vi "FeedbackDecode_DEKAHandCtrl.vi"(1 "RunMode":enum16{"Manual", "Decode"}(ring)) -> ()   [LabVIEW 2020]
uses:
  FeedbackDecode_Globals.vi
  FeedbackDecode_DecodeClust.ctl
  FeedbackDecode_VariablesToString_MDArray.vi
  <vilib>/nican/nican.llb/ncNetAttr.ctl
  <vilib>/nican/nican.llb/CanFrameTimed.ctl
panel:
  in  "DEKAMode":enum16{"Velocity", "Position"}(ring)=enum."Position"
  in  "CtrlMode":T1(array[ring])=[enum."Position", enum."Position", enum."Position", enum."Position", enum."Position", enum."Position", enum."Position", enum."Position", enum."Position", enum."Position", enum."Position", enum."Position"]
  out "MinMax":dbl[][](array[numeric])=[[nan, nan, nan, nan, nan, nan, nan, nan, nan, nan, nan, nan, nan], [nan, nan, nan, nan, nan, nan, nan, nan, nan, nan, nan, nan, nan]]
  in  "Calibrate":bool
  out "LoopCnt":i32
  out "CtrlLoop":dbl(graph)
  in  "ConnDEKA":bool
  in  "MSMSMvnt":dbl[](array[numeric])=[0.0, 0.0, 0.0, 0.0, 0.0, 0.0, 0.0, 0.0, 0.0, 0.0, 0.0, 0.0] min=-1.0 max=1.0
  in  "SensorsRaw":T2={"x241"=[0, 0, 0, 0, 0, 0, 0, 0], "x341"=[0, 0, 0, 0, 0, 0, 0, 0], "x4C2"=[0, 0, 0, 0, 0, 0, 0, 0], "x4AA"=[0, 0, 0, 0, 0, 0, 0, 0], "x4BF"=[0, 0, 0, 0, 0, 0, 0, 0]}
  out "ACITime":dbl(graph)
  out "ACIs":T3[](array[typedef])=[{"Timestamp"=0.0, "ArbitrationId"=528, "IsRemote"=0, "DataLength"=8, "Data"=[0, 0, 0, 0, 0, 0, 0, 0]}, {"Timestamp"=0.0, "ArbitrationId"=529, "IsRemote"=0, "DataLength"=8, "Data"=[0, 0, 0, 0, 0, 0, 0, 0]}, {"Timestamp"=0.0, "ArbitrationId"=530, "IsRemote"=0, "DataLength"=8, "Data"=[0, 0, 0, 0, 0, 0, 0, 0]}, {"Timestamp"=0.0, "ArbitrationId"=531, "IsRemote"=0, "DataLength"=8, "Data"=[0, 0, 0, 0, 0, 0, 0, 0]}] {"Data" format="%.0x"; "ArbitrationId" format="%.0x"; "Timestamp" format="%<%I:%M:%S%3u %p\n%m/%d/%Y>T"}
  out "Sensors":T4
  in  "index":i32
  out "SensorChart":dbl(graph)=12.0
  out "LoopTime":dbl(graph)
  in  "CANConfig":T5={"Start On Open"=enum."TRUE", "Baud Rate"=1000000, "Read Queue Length"=100, "Write Queue Length"=12, "Standard Comparator"=0, "Standard Mask"=0, "Extended Comparator"=0, "Extended Mask"=0} {"Baud Rate" min=5000 max=1333333 step=1; "Extended Mask" format="%.0x"; "Extended Comparator" format="%.0x"; "Standard Mask" format="%.0x"; "Standard Comparator" format="%.0x"; "Write Queue Length" max=1000; "Read Queue Length" max=1000}
  out "Error out":errorcluster {"code" format="%.0x"}
  in  "stop":bool
  in  "CANport":string="CAN0"
  # "ThuPitchUp"
  # "ThuPitchDown"
  # "ThuYawRight"
  # "ThuYawLeft"
  # "IndFlex"
  # "IndExt"
  # "MRPFlex"
  # "MRPExt"
  # "WriPronate"
  # "WriSupinate"
  # "WriExt"
  # "WriFlex"
  # "ModeSelect"
  # "N/A"
  # "N/A"
  # "N/A"
  # "Thumb"
  # "Index"
  # "Middle"
  # "Ring"
  # "Little"
  # "ThumbInt"
  # "IndexInt"
  # "Ring Int"
  # "Little Int"
  # "WristPitch"
  # "WristYaw"
  # "WristRoll"
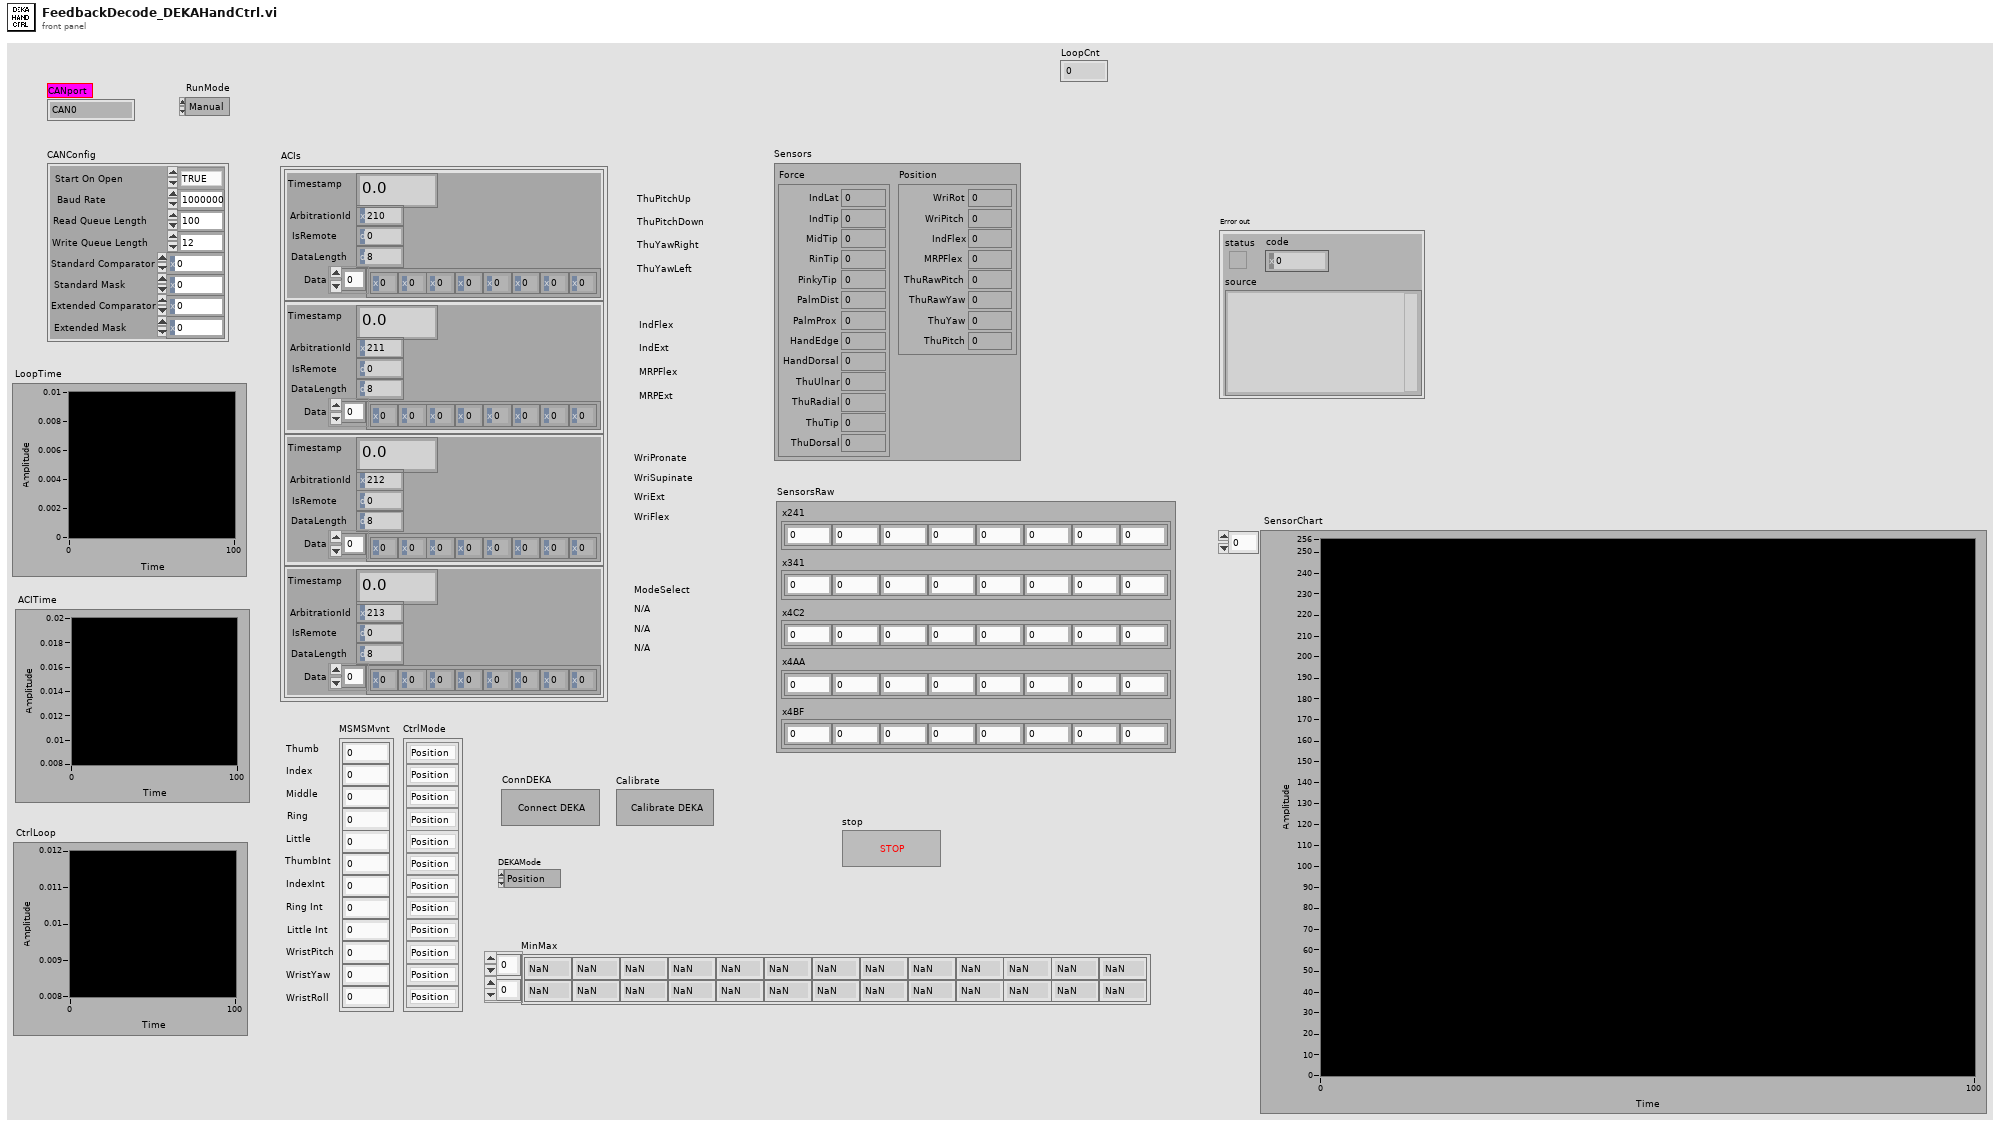
[diagram p1: front panel]
types:
  T1 = enum16{"Position", "Latching", "Leaky", "Velocity"}[]
  T2 = cluster{"x241":u8[], "x341":u8[], "x4C2":u8[], "x4AA":u8[], "x4BF":u8[]}
  T3 = typedef "CanFrameTimed.ctl" = cluster{"Timestamp":dbl, "ArbitrationId":u32, "IsRemote":u8, "DataLength":u8, "Data":u8[]}
  T4 = cluster{"Position":cluster{"WriRot":dbl, "WriPitch":dbl, "IndFlex":dbl, "MRPFlex":dbl, "ThuRawPitch":dbl, "ThuRawYaw":dbl, "ThuYaw":dbl, "ThuPitch":dbl}, "Force":cluster{"IndLat":dbl, "IndTip":dbl, "MidTip":dbl, "RinTip":dbl, "PinkyTip":dbl, "PalmDist":dbl, "PalmProx":dbl, "HandEdge":dbl, "HandDorsal":dbl, "ThuUlnar":dbl, "ThuRadial":dbl, "ThuTip":dbl, "ThuDorsal":dbl}}
  T5 = typedef "ncNetAttr.ctl" = cluster{"Start On Open":enum32{"FALSE", "TRUE"}, "Baud Rate":u32, "Read Queue Length":u32, "Write Queue Length":u32, "Standard Comparator":u32, "Standard Mask":u32, "Extended Comparator":u32, "Extended Mask":u32}
  T6 = typedef "xobjhandle.ctl" = u32
  T7 = enum16{"Position", "Latching", "Leaky", "Velocity"}
  T8 = typedef "FeedbackDecode_DecodeClust.ctl" = cluster{"TrainParams":cluster{"Lag":dbl, "KernelWidth":dbl, "TargRad":dbl}, "Kinematics":cluster{"Thumb":dbl, "Index":dbl, "Middle":dbl, "Ring":dbl, "Little":dbl, "ThumbInt":dbl, "IndexInt":dbl, "RingInt":dbl, "LittleInt":dbl, "Wrist":dbl, "WristYaw":dbl, "WristRoll":dbl}, "CtrlButtons":cluster{"AcqTraining":bool, "ApplyBaseline":bool, "ApplyTraining":bool, "LoadTrainFile":bool, "CAR":bool, "NIPSpikes":bool, "AcqBaseline":bool, "Stop":bool, "ResetTrial":bool, "CalDEKA":bool, "HideSphrs":bool, "StartTrials":bool, "AutoPop":bool, "ResetVRE":bool, "StopVRE":bool, "AcqCAR":bool, "ConARD":bool, "DEKARestart":bool, "ConnDEKA":bool}, "CompID":cluster{"LV":cluster{"Name":string, "IP":string}, "ML":cluster{"Name":string, "IP":string}}, "KMvntClust":cluster{"KGain":sgl[][], "KMvnts":cluster{"Thumb":bool, "Index":bool, "Middle":bool, "Ring":bool, "Little":bool, "ThumbInt":bool, "IndexInt":bool, "RingInt":bool, "LittleInt":bool, "WristPitch":bool, "WristYaw":bool, "WristRoll":bool}, "KThresh":sgl[][], "CtrlMode":enum16{"Position", "Latching", "Leaky", "Velocity"}[], "CtrlSpd":sgl[]}, "ClearUEA":bool, "Targets":cluster{"Thumb":dbl, "Index":dbl, "Middle":dbl, "Ring":dbl, "Little":dbl, "ThumbInt":dbl, "IndexInt":dbl, "RingInt":dbl, "LittleInt":dbl, "Wrist":dbl, "WristYaw":dbl, "WristRoll":dbl}, "KUEAArray":cluster{"Boolean 1":bool, "Boolean 2":bool, "Boolean 3":bool, "Boolean 4":bool, "Boolean 5":bool, "Boolean 6":bool, "Boolean 7":bool, "Boolean 8":bool, "Boolean 9":bool, "Boolean 10":bool, "Boolean 11":bool, "Boolean 12":bool, "Boolean 13":bool, "Boolean 14":bool, "Boolean 15":bool, "Boolean 16":bool, "Boolean 17":bool, "Boolean 18":bool, "Boolean 19":bool, "Boolean 20":bool, "Boolean 21":bool, "Boolean 22":bool, "Boolean 23":bool, "Boolean 24":bool, "Boolean 25":bool, "Boolean 26":bool, "Boolean 27":bool, "Boolean 28":bool, "Boolean 29":bool, "Boolean 30":bool, "Boolean 31":bool, "Boolean 32":bool, "Boolean 33":bool, "Boolean 34":bool, "Boolean 35":bool, "Boolean 36":bool, "Boolean 37":bool, "Boolean 38":bool, "Boolean 39":bool, "Boolean 40":bool, "Boolean 41":bool, "Boolean 42":bool, "Boolean 43":bool, "Boolean 44":bool, "Boolean 45":bool, "Boolean 46":bool, "Boolean 47":bool, "Boolean 48":bool, "Boolean 49":bool, "Boolean 50":bool, "Boolean 51":bool, "Boolean 52":bool, "Boolean 53":bool, "Boolean 54":bool, "Boolean 55":bool, "Boolean 56":bool, "Boolean 57":bool, "Boolean 58":bool, "Boolean 59":bool, "Boolean 60":bool, "Boolean 61":bool, "Boolean 62":bool, "Boolean 63":bool, "Boolean 64":bool, "Boolean 65":bool, "Boolean 66":bool, "Boolean 67":bool, "Boolean 68":bool, "Boolean 69":bool, "Boolean 70":bool, "Boolean 71":bool, "Boolean 72":bool, "Boolean 73":bool, "Boolean 74":bool, "Boolean 75":bool, "Boolean 76":bool, "Boolean 77":bool, "Boolean 78":bool, "Boolean 79":bool, "Boolean 80":bool, "Boolean 81":bool, "Boolean 82":bool, "Boolean 83":bool, "Boolean 84":bool, "Boolean 85":bool, "Boolean 86":bool, "Boolean 87":bool, "Boolean 88":bool, "Boolean 89":bool, "Boolean 90":bool, "Boolean 91":bool, "Boolean 92":bool, "Boolean 93":bool, "Boolean 94":bool, "Boolean 95":bool, "Boolean 96":bool, "Boolean 97":bool, "Boolean 98":bool, "Boolean 99":bool, "Boolean 100":bool}[], "ReTrain":bool, "TargDist":dbl[], "State":enum16{"Initialize", "Acquire Start", "Acquire Response", "Finalize"}, "KalmanType":enum16{"Standard", "Mean", "Refit", "LinSVReg", "NonLinSVReg", "PCA", "DWPRR", "AdaptKF", "NN", "NN_python", "AdaptKF2", "KF_Short_Goal"}, "EventStr":string, "SelElect":dbl, "KinSrc":enum16{"Off", "Training", "Decode", "COB", "LEAP"}, "HoverElect":dbl, "RasterWin":dbl, "WfCnt":dbl, "ClearWfs":bool, "ApplyThresh":bool, "ThreshVal":dbl, "ThreshMode":enum16{"RMS Single", "RMS All", "RMS Auto", "Volt Single", "Volt All"}, "DataFolder":string, "ClearEMG":bool, "KEMGClust":cluster{"Boolean 92":bool, "Boolean 82":bool, "Boolean 72":bool, "Boolean 62":bool, "Boolean 52":bool, "Boolean 42":bool, "Boolean 32":bool, "Boolean 22":bool, "Boolean 12":bool, "Boolean 2":bool, "Boolean 93":bool, "Boolean 83":bool, "Boolean 73":bool, "Boolean 63":bool, "Boolean 53":bool, "Boolean 43":bool, "Boolean 33":bool, "Boolean 23":bool, "Boolean 13":bool, "Boolean 3":bool, "Boolean 94":bool, "Boolean 84":bool, "Boolean 74":bool, "Boolean 64":bool, "Boolean 54":bool, "Boolean 44":bool, "Boolean 34":bool, "Boolean 24":bool, "Boolean 14":bool, "Boolean 4":bool, "Boolean 95":bool, "Boolean 85":bool, "Boolean 75":bool, "Boolean 65":bool, "Boolean 55":bool, "Boolean 45":bool, "Boolean 35":bool, "Boolean 25":bool, "Boolean 15":bool, "Boolean 5":bool, "Boolean 96":bool, "Boolean 86":bool, "Boolean 76":bool, "Boolean 66":bool, "Boolean 56":bool, "Boolean 46":bool, "Boolean 36":bool, "Boolean 26":bool, "Boolean 16":bool, "Boolean 6":bool, "Boolean 97":bool, "Boolean 87":bool, "Boolean 77":bool, "Boolean 67":bool, "Boolean 57":bool, "Boolean 47":bool, "Boolean 37":bool, "Boolean 27":bool, "Boolean 17":bool, "Boolean 7":bool, "Boolean 98":bool, "Boolean 88":bool, "Boolean 78":bool, "Boolean 68":bool, "Boolean 58":bool, "Boolean 48":bool, "Boolean 38":bool, "Boolean 28":bool, "Boolean 18":bool, "Boolean 8":bool, "Boolean 99":bool, "Boolean 89":bool, "Boolean 79":bool, "Boolean 69":bool, "Boolean 59":bool, "Boolean 49":bool, "Boolean 39":bool, "Boolean 29":bool, "Boolean 19":bool, "Boolean 9":bool}, "EvntFlag":bool, "FillUEA":bool, "FillEMG":bool, "FillMvnts":bool, "BadUEAElects":dbl[], "KEMGExtra":dbl[], "AllPairs":bool, "AutoThresh":dbl, "BadEMGChans":dbl[], "LinkedDOF":string, "AutoPopType":enum16{"Standard", "Stepwise", "Gram"}, "CARType":enum16{"Standard", "NN"}, "*Map":enum16{"pNeural/pEMG", "pNeural/aEMG", "aNeural/pEMG", "aNeural/aEMG", "N2021/pEMG"}, "GainFill":dbl, "ThreshFill":dbl, "TestType":enum16{"MSMS", "Bakeoff11", "Bakeoff21", "Bakeoff31", "Bakeoff32", "Bakeoff32_Ball", "Bakeoff32_Checkers", "Bakeoff32_Pen", "FragileBlock"}, "Outcome":enum16{"---", "Success", "Failure"}, "TrialCnt":dbl[][], "ClearTrials":bool, "Log10":bool, "KDFFile":string, "LimitExt":bool, "*Prosthesis":enum16{"MaleRight", "MaleLeft"}, "StartML":bool, "StartMLAux":bool, "StartRec":bool, "DynaThr":bool, "ModeFill":enum16{"Position", "Latching", "Leaky", "Velocity"}, "SpdFill":dbl, "DEKAMode":enum16{"Velocity", "Position"}, "FreeParam":dbl, "GoalNoise":dbl, "Load NN":bool, "ExportTrain":bool, "NumComp":enum16{"1 Computer", "2 Computers"}, "DataDir":string, "BuildDir":string, "LatchingFilter":bool, "Trigger":bool, "StartARD":bool, "StartTaska":bool, "StartTaskaSens":bool}
  T9 = enum16{"Initialize", "Wait", "BuildInitStr", "BuildKalmanStr", "BuildStimStr", "BuildEMGStr", "GetEvent", "SendEvent", "ContIO", "LoadTrainFile", "CopyTraining", "Close"}
  T10 = cluster{"IndLat":dbl, "IndTip":dbl, "MidTip":dbl, "RinTip":dbl, "PinkyTip":dbl, "PalmDist":dbl, "PalmProx":dbl, "HandEdge":dbl, "HandDorsal":dbl, "ThuUlnar":dbl, "ThuRadial":dbl, "ThuTip":dbl, "ThuDorsal":dbl}
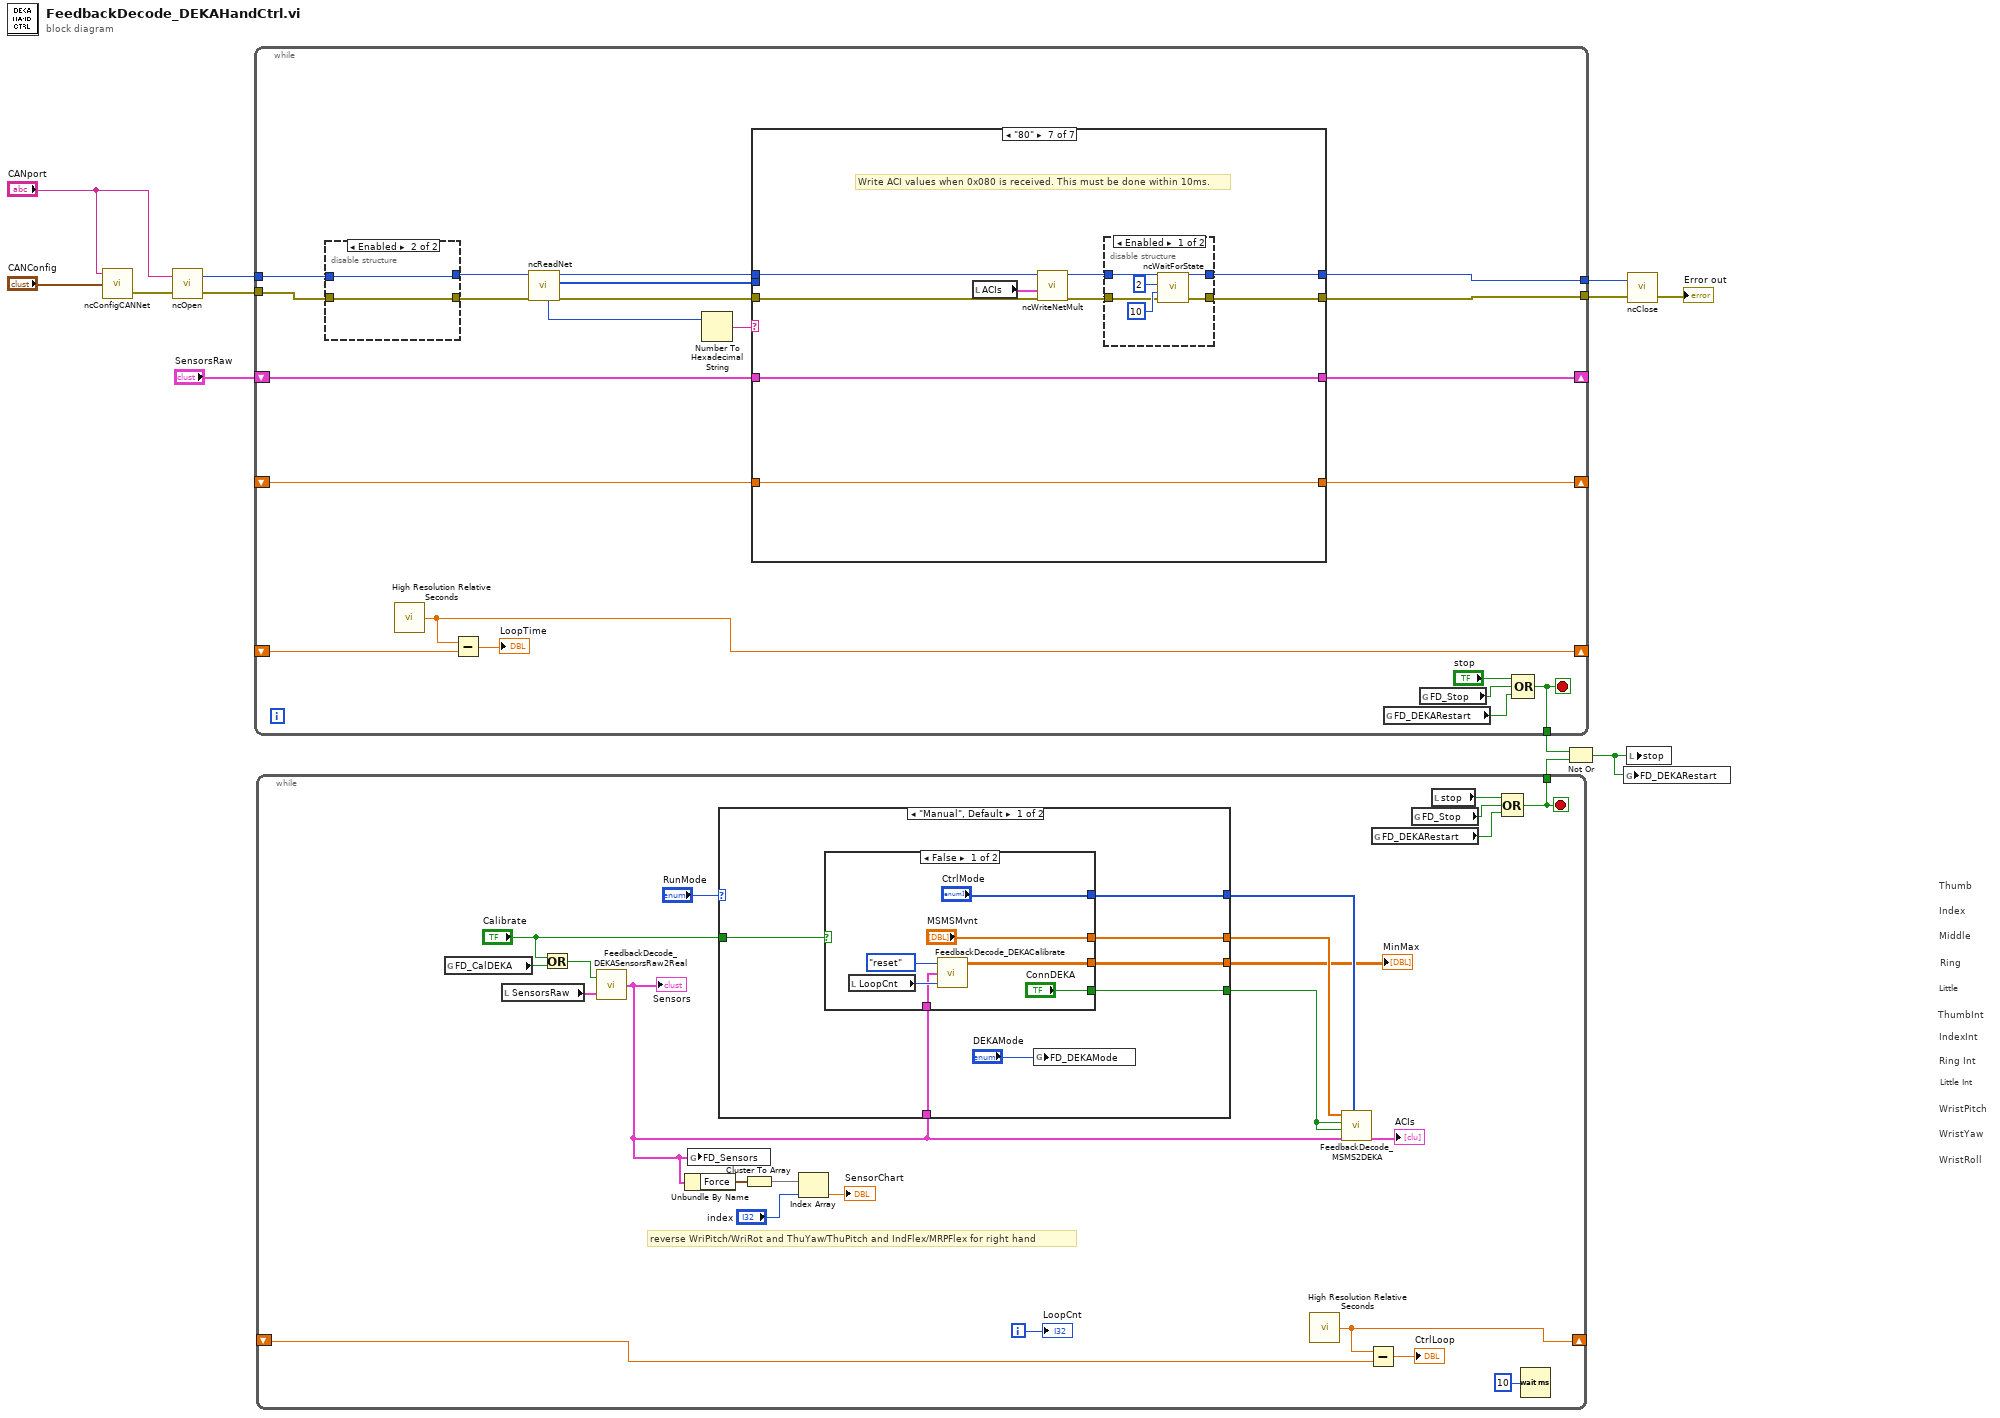
[diagram p0: block diagram]
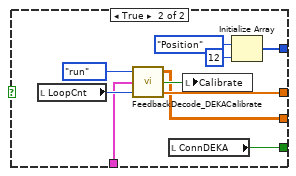
[diagram p2: hidden frame]
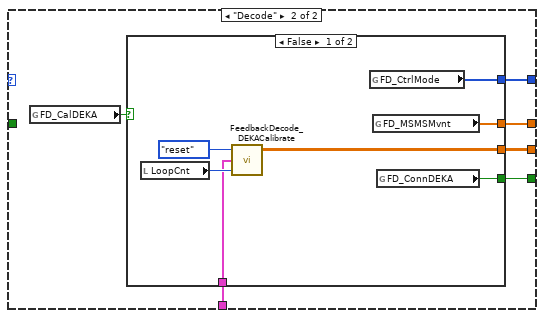
[diagram p3: hidden frame]
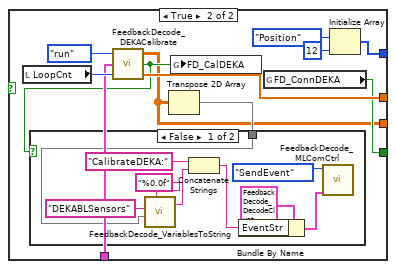
[diagram p4: hidden frame]
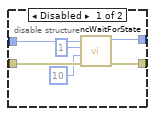
[diagram p6: hidden frame]
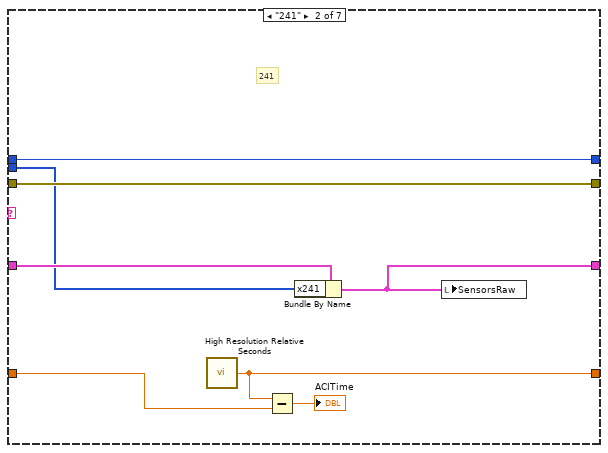
[diagram p8: hidden frame]
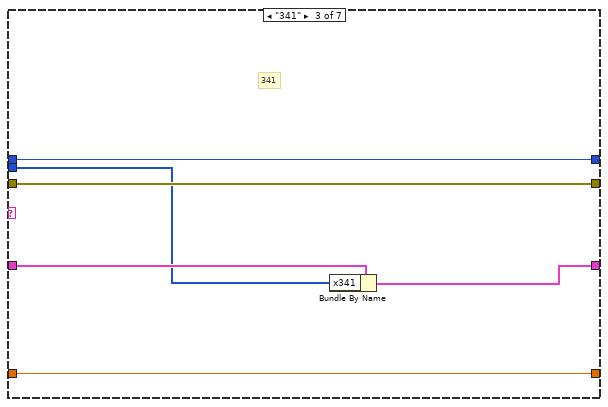
[diagram p9: hidden frame]
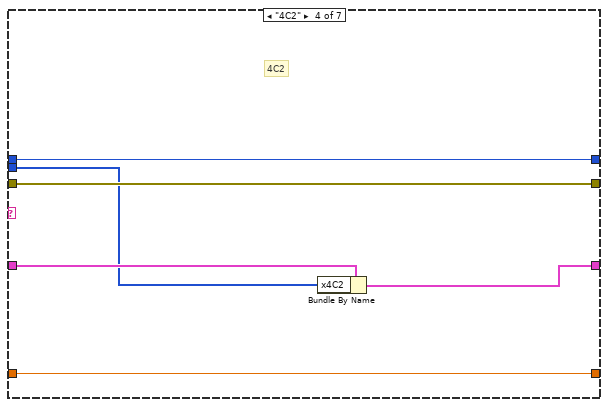
[diagram p10: hidden frame]
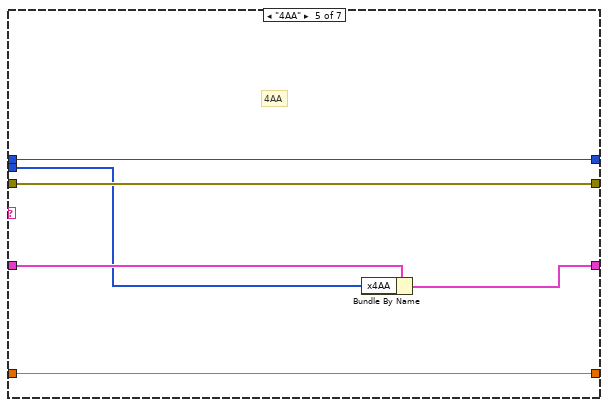
[diagram p11: hidden frame]
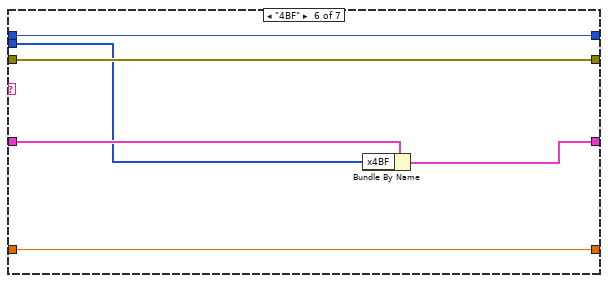
[diagram p12: hidden frame]
diagram:
  # "Little Int"
  # "WristRoll"
  # "WristYaw"
  # "WristPitch"
  # "Ring Int"
  # "IndexInt"
  # "ThumbInt"
  # "Little"
  # "Ring"
  # "Middle"
  # "Index"
  # "Thumb"
  n1 = call <vilib>:"ncConfigCANNet.vi"("CAN Network Interface Config"="CANConfig", "ObjName"="CANport") -> ("Error out"=w11:errorcluster)  [unwired: 3 in]
  n2 = call <vilib>:"ncOpen.vi"("Error in"=w11, "ObjName"="CANport") -> ("Error out"=w5:errorcluster, "ObjHandle out"=w6:T6)
  n3 = while {
    tunnel: w5 -> [w34]
    tunnel: [w25] -> w10
    tunnel: w6 -> [w32]
    tunnel: [w28] -> w8
    shift-right: [w29] -> _
    shift-left: _ -> [w30]
    shift-right: [w23] -> _
    shift-left: "SensorsRaw" -> [w24]
    shift-right: [w17] -> _
    shift-left: _ -> [w18]
    tunnel: [w14] -> w4
    stop <- w14 stop-if-true
    n4 = disable-structure shown="Enabled" {
      disable-tunnel: w34 -> [w40 w41]
      disable-tunnel: [w39 w41] -> w33
      disable-tunnel: w32 -> [w38 w42]
      disable-tunnel: [w37 w42] -> w31
      frame Disabled {
        n5 = call <vilib>:"ncWaitForState.vi"("Error in"=w40, "Timeout"=u32 10, "DesiredState"=u32 1 ("state"), "ObjHandle in"=w38) -> ("Error out"=w39:errorcluster, "ObjHandle out"=w37:T6)  [unwired: 1 out]
      }
      frame Enabled {
      }
    }
    n6 = call <vilib>:"High Resolution Relative Seconds.vi"() -> ("relative seconds"=w29:dbl)
    n7 = Subtract(x=w29, y=w30) -> (x-y=→"LoopTime":dbl)
    n8 = call <vilib>:"ncReadNet.vi"("ObjHandle in"=w31, "Error in"=w33) -> ("ArbitrationId"=w20:u32, "ObjHandle out"=w27:T6, "Data"=w19:u8[], "Error out"=w26:errorcluster)  [unwired: 2 in, 3 out]
    n9 = Number To Hexadecimal String(2:w20) -> (0:w21:string)  [unwired: 1 in]
    n10 = case shown="\"80\"" w21 {
      tunnel: [w46 w54 w60 w66 w72 w78 w82] -> w28
      tunnel: w27 -> [w46 w54 w60 w66 w72 w78 w87]
      tunnel: w19 -> [_ w51 w55 w61 w67 w73 _]
      tunnel: w26 -> [w45 w53 w59 w65 w71 w77 w86]
      tunnel: [w45 w53 w59 w65 w71 w77 w83] -> w25
      tunnel: w24 -> [w44 w52 w58 w64 w70 w76 w80]
      tunnel: [w44 w50 w57 w63 w69 w75 w80] -> w23
      tunnel: w18 -> [w43 w48 w56 w62 w68 w74 w79]
      tunnel: [w43 w47 w56 w62 w68 w74 w79] -> w17
      frame "0", Default {
      }
      frame "241" {
        # "241"
        n11 = call <vilib>:"High Resolution Relative Seconds.vi"() -> ("relative seconds"=w47:dbl)
        n12 = Subtract(x=w47, y=w48) -> (x-y=→"ACITime":dbl)
        n13 = Bundle By Name(cluster=w52, "x241"=w51) -> (w50:T2)
        n14 = local write "SensorsRaw"(w50) -> ()
      }
      frame "341" {
        # "341"
        n15 = Bundle By Name(cluster=w58, "x341"=w55) -> (w57:T2)
      }
      frame "4C2" {
        # "4C2"
        n16 = Bundle By Name(cluster=w64, "x4C2"=w61) -> (w63:T2)
      }
      frame "4AA" {
        # "4AA"
        n17 = Bundle By Name(cluster=w70, "x4AA"=w67) -> (w69:T2)
      }
      frame "4BF" {
        n18 = Bundle By Name(cluster=w76, "x4BF"=w73) -> (w75:T2)
      }
      frame "80" {
        # "Write ACI values when 0x080 is received. This must be done within 10ms."
        n19 = local read "ACIs"() -> (w81:T3[])
        n20 = call <vilib>:"ncWriteNetMult.vi"("Error in"=w86, "Data"=w81, "ObjHandle in"=w87) -> ("Error out"=w84:errorcluster, "ObjHandle out"=w85:T6)  [unwired: 7 in]
        n21 = disable-structure shown="Enabled" {
          disable-tunnel: w85 -> [w91 w95]
          disable-tunnel: w84 -> [w90 w94]
          disable-tunnel: [w89 w94] -> w83
          disable-tunnel: [w88 w95] -> w82
          frame Enabled {
            n22 = call <vilib>:"ncWaitForState.vi"("Error in"=w90, "Timeout"=u32 10, "DesiredState"=u32 2 ("state"), "ObjHandle in"=w91) -> ("Error out"=w89:errorcluster, "ObjHandle out"=w88:T6)  [unwired: 1 out]
          }
          frame Disabled {
          }
        }
      }
    }
    n23 = global read "FeedbackDecode_Globals.vi" "FD_DEKARestart"() -> (w13:bool)
    n24 = global read "FeedbackDecode_Globals.vi" "FD_Stop"() -> (w15:bool)
    n25 = Compound Arithmetic op=OR("stop", w15, w13) -> (w14:bool)
  }
  n26 = while {
    tunnel: [w112] -> w3
    shift-right: [w107] -> _
    shift-left: _ -> [w108]
    i -> [w102]
    stop <- w112 stop-if-true
    # "reverse WriPitch/WriRot and ThuYaw/ThuPitch and IndFlex/MRPFlex for right hand"
    n27 = global read "FeedbackDecode_Globals.vi" "FD_CalDEKA"() -> (w98:bool)
    n28 = local read "SensorsRaw"() -> (w100:T2)
    n29 = Or(x="Calibrate", y=w98) -> (x .or. y?=w96:bool)
    n30 = call "FeedbackDecode_DEKASensorsRaw2Real.vi"("SensorsRaw"=w100, "Calibration?"=w96) -> ("Sensors"=w99:T4)
    "Sensors" <- w99
    n31 = Unbundle By Name(w99) -> ("Force"=w117:T10)
    n32 = global write "FeedbackDecode_Globals.vi" "FD_Sensors"(w99) -> ()
    n33 = case shown="\"Manual\", Default" "RunMode" {
      tunnel: [w123 w148] -> w106
      tunnel: [w125 w149] -> w111
      tunnel: [w124 w147] -> w105
      tunnel: w99 -> [w126 w146]
      tunnel: [w122 w144] -> w101
      tunnel: "Calibrate" -> [w121 _]
      frame "Manual", Default {
        n34 = case shown="False" w121 {
          tunnel: w126 -> [w130 w141]
          tunnel: ["MSMSMvnt" w140] -> w125
          tunnel: ["CtrlMode" w134] -> w124
          tunnel: ["ConnDEKA" w139] -> w123
          tunnel: [w128 w137] -> w122
          frame False {
            n35 = local read "LoopCnt"() -> (w131:i32)
            n36 = call "FeedbackDecode_DEKACalibrate.vi"("LoopCnt"=w131, "SensorsIn"=w130, "Mode"=enum16{"reset", "run"}."reset") -> ("MinMax"=w128:dbl[][])  [unwired: 2 out]
          }
          frame True {
            n37 = local read "LoopCnt"() -> (w142:i32)
            n38 = call "FeedbackDecode_DEKACalibrate.vi"("LoopCnt"=w142, "SensorsIn"=w141, "Mode"=enum16{"reset", "run"}."run") -> ("MSMSMvnt"=w140:dbl[], "Status"=w138:bool, "MinMax"=w137:dbl[][])
            n39 = local read "ConnDEKA"() -> (w139:bool)
            n40 = local write "Calibrate"(w138) -> ()
            n41 = Initialize Array(T7."Position" ("DEKACtrlMode"), 12 ("dimension size")) -> (w134:T1)
          }
        }
        n42 = global write "FeedbackDecode_Globals.vi" "FD_DEKAMode"("DEKAMode") -> ()
      }
      frame "Decode" {
        n43 = global read "FeedbackDecode_Globals.vi" "FD_CalDEKA"() -> (w145:bool)
        n44 = case shown="False" w145 {
          tunnel: [w156 w165] -> w149
          tunnel: [w155 w164] -> w148
          tunnel: [w154 w157] -> w147
          tunnel: w146 -> [w151 w163]
          tunnel: [w150 w160] -> w144
          frame False {
            n45 = local read "LoopCnt"() -> (w152:i32)
            n46 = call "FeedbackDecode_DEKACalibrate.vi"("LoopCnt"=w152, "SensorsIn"=w151, "Mode"=enum16{"reset", "run"}."reset") -> ("MinMax"=w150:dbl[][])  [unwired: 2 out]
            n47 = global read "FeedbackDecode_Globals.vi" "FD_CtrlMode"() -> (w154:T1)
            n48 = global read "FeedbackDecode_Globals.vi" "FD_MSMSMvnt"() -> (w156:dbl[])
            n49 = global read "FeedbackDecode_Globals.vi" "FD_ConnDEKA"() -> (w155:bool)
          }
          frame True {
            n50 = local read "LoopCnt"() -> (w166:i32)
            n51 = call "FeedbackDecode_DEKACalibrate.vi"("LoopCnt"=w166, "SensorsIn"=w163, "Mode"=enum16{"reset", "run"}."run") -> ("MSMSMvnt"=w165:dbl[], "Status"=w162:bool, "MinMax"=w160:dbl[][])
            n52 = Transpose 2D Array(2D array=w160) -> (transposed array=w161:dbl[][])
            n53 = case shown="False" w162 {
              tunnel: w161 -> [w169 _]
              frame False {
                n54 = call-poly "FeedbackDecode_VariablesToString.vi"("Format"="%0.0f", "ValueIn"=w169, "FieldName"="DEKABLSensors" ("EventStr")) -> ("StringOut"=w173:string)  [unwired: 4 in]
                n55 = Concatenate Strings("CalibrateDEKA:" ("EventStr"), w173) -> (w170:string)
                n56 = Bundle By Name(cluster=T8 {"TrainParams"={"Lag"=0.0, "KernelWidth"=0.3, "TargRad"=0.15}, "Kinematics"={"Thumb"=0.0, "Index"=0.0, "Middle"=0.0, "Ring"=0.0, "Little"=0.0, "ThumbInt"=0.0, "IndexInt"=0.0, "RingInt"=0.0, "LittleInt"=0.0, "Wrist"=0.0, "WristYaw"=0.0, "WristRoll"=0.0}, "CtrlButtons"={"AcqTraining"=FALSE, "ApplyBaseline"=FALSE, "ApplyTraining"=FALSE, "LoadTrainFile"=FALSE, "CAR"=FALSE, "NIPSpikes"=FALSE, "AcqBaseline"=FALSE, "Stop"=FALSE, "ResetTrial"=FALSE, "CalDEKA"=FALSE, "HideSphrs"=FALSE, "StartTrials"=FALSE, "AutoPop"=FALSE, "ResetVRE"=FALSE, "StopVRE"=FALSE, "AcqCAR"=FALSE, "ConARD"=FALSE, "DEKARestart"=FALSE, "ConnDEKA"=FALSE}, "CompID"={"LV"={"Name"="PNILABVIEW", "IP"="155.100.90.215"}, "ML"={"Name"="PNIMATLAB", "IP"="155.100.91.231"}}, "KMvntClust"={"KGain"=[[1.0, 1.0, -1.0, 1.0], [1.0, 1.0, -1.0, 1.0], [1.0, 1.0, -1.0, 1.0], [1.0, 1.0, -1.0, 1.0], [1.0, 1.0, -1.0, 1.0], [1.0, 1.0, -1.0, 1.0], [1.0, 1.0, -1.0, 1.0], [1.0, 1.0, -1.0, 1.0], [1.0, 1.0, -1.0, 1.0], [1.0, 1.0, -1.0, 1.0], [1.0, 1.0, -1.0, 1.0], [1.0, 1.0, -1.0, 1.0]], "KMvnts"={"Thumb"=FALSE, "Index"=FALSE, "Middle"=FALSE, "Ring"=FALSE, "Little"=FALSE, "ThumbInt"=FALSE, "IndexInt"=FALSE, "RingInt"=FALSE, "LittleInt"=FALSE, "WristPitch"=FALSE, "WristYaw"=FALSE, "WristRoll"=FALSE}, "KThresh"=[[0.2, 0.2, -1.0, 1.0], [0.2, 0.2, -1.0, 1.0], [0.2, 0.2, -1.0, 1.0], [0.2, 0.2, -1.0, 1.0], [0.2, 0.2, -1.0, 1.0], [0.2, 0.2, -1.0, 1.0], [0.2, 0.2, -1.0, 1.0], [0.2, 0.2, -1.0, 1.0], [0.2, 0.2, -1.0, 1.0], [0.2, 0.2, -1.0, 1.0], [0.2, 0.2, -1.0, 1.0], [0.2, 0.2, -1.0, 1.0]], "CtrlMode"=[], "CtrlSpd"=[]}, "ClearUEA"=FALSE, "Targets"={"Thumb"=0.0, "Index"=0.0, "Middle"=0.0, "Ring"=0.0, "Little"=0.0, "ThumbInt"=0.0, "IndexInt"=0.0, "RingInt"=0.0, "LittleInt"=0.0, "Wrist"=0.0, "WristYaw"=0.0, "WristRoll"=0.0}, "KUEAArray"=[{"Boolean 1"=FALSE, "Boolean 2"=FALSE, "Boolean 3"=FALSE, "Boolean 4"=FALSE, "Boolean 5"=FALSE, "Boolean 6"=FALSE, "Boolean 7"=FALSE, "Boolean 8"=FALSE, "Boolean 9"=FALSE, "Boolean 10"=FALSE, "Boolean 11"=FALSE, "Boolean 12"=FALSE, "Boolean 13"=FALSE, "Boolean 14"=FALSE, "Boolean 15"=FALSE, "Boolean 16"=FALSE, "Boolean 17"=FALSE, "Boolean 18"=FALSE, "Boolean 19"=FALSE, "Boolean 20"=FALSE, "Boolean 21"=FALSE, "Boolean 22"=FALSE, "Boolean 23"=FALSE, "Boolean 24"=FALSE, "Boolean 25"=FALSE, "Boolean 26"=FALSE, "Boolean 27"=FALSE, "Boolean 28"=FALSE, "Boolean 29"=FALSE, "Boolean 30"=FALSE, "Boolean 31"=FALSE, "Boolean 32"=FALSE, "Boolean 33"=FALSE, "Boolean 34"=FALSE, "Boolean 35"=FALSE, "Boolean 36"=FALSE, "Boolean 37"=FALSE, "Boolean 38"=FALSE, "Boolean 39"=FALSE, "Boolean 40"=FALSE, "Boolean 41"=FALSE, "Boolean 42"=FALSE, "Boolean 43"=FALSE, "Boolean 44"=FALSE, "Boolean 45"=FALSE, "Boolean 46"=FALSE, "Boolean 47"=FALSE, "Boolean 48"=FALSE, "Boolean 49"=FALSE, "Boolean 50"=FALSE, "Boolean 51"=FALSE, "Boolean 52"=FALSE, "Boolean 53"=FALSE, "Boolean 54"=FALSE, "Boolean 55"=FALSE, "Boolean 56"=FALSE, "Boolean 57"=FALSE, "Boolean 58"=FALSE, "Boolean 59"=FALSE, "Boolean 60"=FALSE, "Boolean 61"=FALSE, "Boolean 62"=FALSE, "Boolean 63"=FALSE, "Boolean 64"=FALSE, "Boolean 65"=FALSE, "Boolean 66"=FALSE, "Boolean 67"=FALSE, "Boolean 68"=FALSE, "Boolean 69"=FALSE, "Boolean 70"=FALSE, "Boolean 71"=FALSE, "Boolean 72"=FALSE, "Boolean 73"=FALSE, "Boolean 74"=FALSE, "Boolean 75"=FALSE, "Boolean 76"=FALSE, "Boolean 77"=FALSE, "Boolean 78"=FALSE, "Boolean 79"=FALSE, "Boolean 80"=FALSE, "Boolean 81"=FALSE, "Boolean 82"=FALSE, "Boolean 83"=FALSE, "Boolean 84"=FALSE, "Boolean 85"=FALSE, "Boolean 86"=FALSE, "Boolean 87"=FALSE, "Boolean 88"=FALSE, "Boolean 89"=FALSE, "Boolean 90"=FALSE, "Boolean 91"=FALSE, "Boolean 92"=FALSE, "Boolean 93"=FALSE, "Boolean 94"=FALSE, "Boolean 95"=FALSE, "Boolean 96"=FALSE, "Boolean 97"=FALSE, "Boolean 98"=FALSE, "Boolean 99"=FALSE, "Boolean 100"=FALSE}, {"Boolean 1"=FALSE, "Boolean 2"=FALSE, "Boolean 3"=FALSE, "Boolean 4"=FALSE, "Boolean 5"=FALSE, "Boolean 6"=FALSE, "Boolean 7"=FALSE, "Boolean 8"=FALSE, "Boolean 9"=FALSE, "Boolean 10"=FALSE, "Boolean 11"=FALSE, "Boolean 12"=FALSE, "Boolean 13"=FALSE, "Boolean 14"=FALSE, "Boolean 15"=FALSE, "Boolean 16"=FALSE, "Boolean 17"=FALSE, "Boolean 18"=FALSE, "Boolean 19"=FALSE, "Boolean 20"=FALSE, "Boolean 21"=FALSE, "Boolean 22"=FALSE, "Boolean 23"=FALSE, "Boolean 24"=FALSE, "Boolean 25"=FALSE, "Boolean 26"=FALSE, "Boolean 27"=FALSE, "Boolean 28"=FALSE, "Boolean 29"=FALSE, "Boolean 30"=FALSE, "Boolean 31"=FALSE, "Boolean 32"=FALSE, "Boolean 33"=FALSE, "Boolean 34"=FALSE, "Boolean 35"=FALSE, "Boolean 36"=FALSE, "Boolean 37"=FALSE, "Boolean 38"=FALSE, "Boolean 39"=FALSE, "Boolean 40"=FALSE, "Boolean 41"=FALSE, "Boolean 42"=FALSE, "Boolean 43"=FALSE, "Boolean 44"=FALSE, "Boolean 45"=FALSE, "Boolean 46"=FALSE, "Boolean 47"=FALSE, "Boolean 48"=FALSE, "Boolean 49"=FALSE, "Boolean 50"=FALSE, "Boolean 51"=FALSE, "Boolean 52"=FALSE, "Boolean 53"=FALSE, "Boolean 54"=FALSE, "Boolean 55"=FALSE, "Boolean 56"=FALSE, "Boolean 57"=FALSE, "Boolean 58"=FALSE, "Boolean 59"=FALSE, "Boolean 60"=FALSE, "Boolean 61"=FALSE, "Boolean 62"=FALSE, "Boolean 63"=FALSE, "Boolean 64"=FALSE, "Boolean 65"=FALSE, "Boolean 66"=FALSE, "Boolean 67"=FALSE, "Boolean 68"=FALSE, "Boolean 69"=FALSE, "Boolean 70"=FALSE, "Boolean 71"=FALSE, "Boolean 72"=FALSE, "Boolean 73"=FALSE, "Boolean 74"=FALSE, "Boolean 75"=FALSE, "Boolean 76"=FALSE, "Boolean 77"=FALSE, "Boolean 78"=FALSE, "Boolean 79"=FALSE, "Boolean 80"=FALSE, "Boolean 81"=FALSE, "Boolean 82"=FALSE, "Boolean 83"=FALSE, "Boolean 84"=FALSE, "Boolean 85"=FALSE, "Boolean 86"=FALSE, "Boolean 87"=FALSE, "Boolean 88"=FALSE, "Boolean 89"=FALSE, "Boolean 90"=FALSE, "Boolean 91"=FALSE, "Boolean 92"=FALSE, "Boolean 93"=FALSE, "Boolean 94"=FALSE, "Boolean 95"=FALSE, "Boolean 96"=FALSE, "Boolean 97"=FALSE, "Boolean 98"=FALSE, "Boolean 99"=FALSE, "Boolean 100"=FALSE}], "ReTrain"=FALSE, "TargDist"=[0.0, 0.0, 0.0, 0.0, 0.0, 0.0], "State"=enum."Initialize", "KalmanType"=enum."Standard", "EventStr"="", "SelElect"=1.0, "KinSrc"=enum."Training", "HoverElect"=0.0, "RasterWin"=1.0, "WfCnt"=15.0, "ClearWfs"=FALSE, "ApplyThresh"=FALSE, "ThreshVal"=-5.0, "ThreshMode"=enum."RMS Single", "DataFolder"="00000000-000000", "ClearEMG"=FALSE, "KEMGClust"={"Boolean 92"=FALSE, "Boolean 82"=FALSE, "Boolean 72"=FALSE, "Boolean 62"=FALSE, "Boolean 52"=FALSE, "Boolean 42"=FALSE, "Boolean 32"=FALSE, "Boolean 22"=FALSE, "Boolean 12"=FALSE, "Boolean 2"=FALSE, "Boolean 93"=FALSE, "Boolean 83"=FALSE, "Boolean 73"=FALSE, "Boolean 63"=FALSE, "Boolean 53"=FALSE, "Boolean 43"=FALSE, "Boolean 33"=FALSE, "Boolean 23"=FALSE, "Boolean 13"=FALSE, "Boolean 3"=FALSE, "Boolean 94"=FALSE, "Boolean 84"=FALSE, "Boolean 74"=FALSE, "Boolean 64"=FALSE, "Boolean 54"=FALSE, "Boolean 44"=FALSE, "Boolean 34"=FALSE, "Boolean 24"=FALSE, "Boolean 14"=FALSE, "Boolean 4"=FALSE, "Boolean 95"=FALSE, "Boolean 85"=FALSE, "Boolean 75"=FALSE, "Boolean 65"=FALSE, "Boolean 55"=FALSE, "Boolean 45"=FALSE, "Boolean 35"=FALSE, "Boolean 25"=FALSE, "Boolean 15"=FALSE, "Boolean 5"=FALSE, "Boolean 96"=FALSE, "Boolean 86"=FALSE, "Boolean 76"=FALSE, "Boolean 66"=FALSE, "Boolean 56"=FALSE, "Boolean 46"=FALSE, "Boolean 36"=FALSE, "Boolean 26"=FALSE, "Boolean 16"=FALSE, "Boolean 6"=FALSE, "Boolean 97"=FALSE, "Boolean 87"=FALSE, "Boolean 77"=FALSE, "Boolean 67"=FALSE, "Boolean 57"=FALSE, "Boolean 47"=FALSE, "Boolean 37"=FALSE, "Boolean 27"=FALSE, "Boolean 17"=FALSE, "Boolean 7"=FALSE, "Boolean 98"=FALSE, "Boolean 88"=FALSE, "Boolean 78"=FALSE, "Boolean 68"=FALSE, "Boolean 58"=FALSE, "Boolean 48"=FALSE, "Boolean 38"=FALSE, "Boolean 28"=FALSE, "Boolean 18"=FALSE, "Boolean 8"=FALSE, "Boolean 99"=FALSE, "Boolean 89"=FALSE, "Boolean 79"=FALSE, "Boolean 69"=FALSE, "Boolean 59"=FALSE, "Boolean 49"=FALSE, "Boolean 39"=FALSE, "Boolean 29"=FALSE, "Boolean 19"=FALSE, "Boolean 9"=FALSE}, "EvntFlag"=FALSE, "FillUEA"=FALSE, "FillEMG"=FALSE, "FillMvnts"=FALSE, "BadUEAElects"=[], "KEMGExtra"=[], "AllPairs"=FALSE, "AutoThresh"=0.4, "BadEMGChans"=[], "LinkedDOF"="{}", "AutoPopType"=enum."Standard", "CARType"=enum."Standard", "*Map"=enum."pNeural/pEMG", "GainFill"=1.0, "ThreshFill"=1.0, "TestType"=enum."MSMS", "Outcome"=enum."---", "TrialCnt"=[], "ClearTrials"=FALSE, "Log10"=FALSE, "KDFFile"="{}", "LimitExt"=FALSE, "*Prosthesis"=enum."MaleLeft", "StartML"=FALSE, "StartMLAux"=FALSE, "StartRec"=FALSE, "DynaThr"=FALSE, "ModeFill"=enum."Position", "SpdFill"=1.0, "DEKAMode"=enum."Velocity", "FreeParam"=0.4, "GoalNoise"=0.4, "Load NN"=FALSE, "ExportTrain"=FALSE, "NumComp"=enum."2 Computers", "DataDir"="00000000-000000", "BuildDir"="00000000-000000", "LatchingFilter"=FALSE, "Trigger"=FALSE, "StartARD"=FALSE, "StartTaska"=FALSE, "StartTaskaSens"=FALSE} ("DecodeClustIn"), "EventStr"=w170) -> (w176:T8)
                n57 = call "FeedbackDecode_MLComCtrl.vi"("DecodeClustIn"=w176, "Mode"=T9."SendEvent") -> ()  [unwired: 3 in, 3 out]
              }
              frame True {
              }
            }
            n58 = global write "FeedbackDecode_Globals.vi" "FD_CalDEKA"(w162) -> ()
            n59 = global read "FeedbackDecode_Globals.vi" "FD_ConnDEKA"() -> (w164:bool)
            n60 = Initialize Array(T7."Position" ("DEKACtrlMode"), 12 ("dimension size")) -> (w157:T1)
          }
        }
      }
    }
    "MinMax" <- w101
    n61 = Cluster To Array(cluster=w117) -> (array=w118:dbl[])
    n62 = Index Array(array=w118, index="index") -> (element=→"SensorChart":dbl)
    n63 = call <vilib>:"High Resolution Relative Seconds.vi"() -> ("relative seconds"=w107:dbl)
    n64 = call "FeedbackDecode_MSMS2DEKA.vi"("CtrlMode"=w105, "Sensors"=w99, "ConnDEKA"=w106, "ResetPID"=w106, "MSMSMvnt"=w111) -> ("ACIOut"=→"ACIs":T3[])  [unwired: 6 in]
    n65 = Subtract(x=w107, y=w108) -> (x-y=→"CtrlLoop":dbl)
    n66 = global read "FeedbackDecode_Globals.vi" "FD_DEKARestart"() -> (w104:bool)
    n67 = global read "FeedbackDecode_Globals.vi" "FD_Stop"() -> (w113:bool)
    n68 = local read "stop"() -> (w114:bool)
    n69 = Compound Arithmetic op=OR(w114, w113, w104) -> (w112:bool)
    n70 = Wait (ms)(milliseconds to wait=u32 10) -> ()  [unwired: 1 out]
    "LoopCnt" <- w102
  }
  n71 = Not Or(1:w3, 2:w4) -> (0:w1:bool)
  n72 = global write "FeedbackDecode_Globals.vi" "FD_DEKARestart"(w1) -> ()
  n73 = local write "stop"(w1) -> ()
  n74 = call <vilib>:"ncClose.vi"("Error in"=w10, "ObjHandle in"=w8) -> ("Error out"=→"Error out":errorcluster)  [unwired: 1 in]
